vi "init.vi"(8 "error in (no error)":errorcluster, 11 "HP83712B_RF_Generator in":refnum<class "HP83712B_RF_Generator.lvclass">) -> (0 "error out":errorcluster, 3 "HP83712B_RF_Generator out":refnum<class "HP83712B_RF_Generator.lvclass">)   [LabVIEW 2013, in "HP83712B_RF_Generator.lvclass"]
uses:
  HP83712B_RF_Generator.lvclass
  HP83712B_RF_Generator.lvclass/HP83712B_RF_Generator.ctl
  Experiment/Globals.vi
  HP8662A_RF_Generator/HP8662A_RF_Generator.lvclass
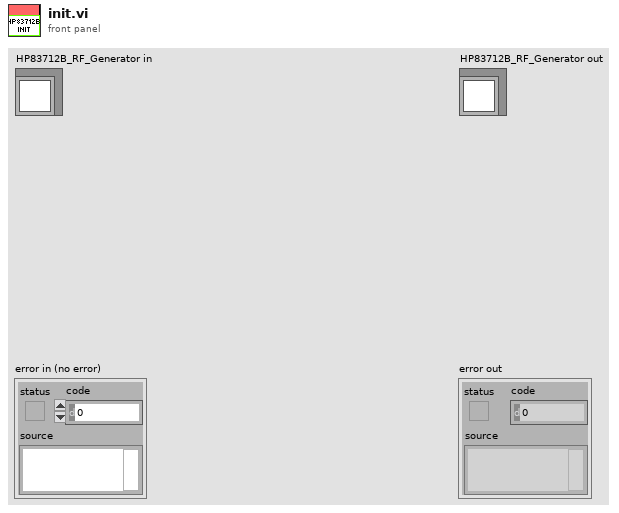
[diagram p1: front panel]
types:
  T1 = typedef "GPIB.lvclass/RF_Generator_settings_array.ctl" = T2[]
  T2 = typedef "GPIB.lvclass/RF_Generator_settings.ctl" = cluster{"Enable":bool, "Description":string, "GPIB channel #":u8, "Frequency (MHz)":dbl, "Power (dBm)":dbl}
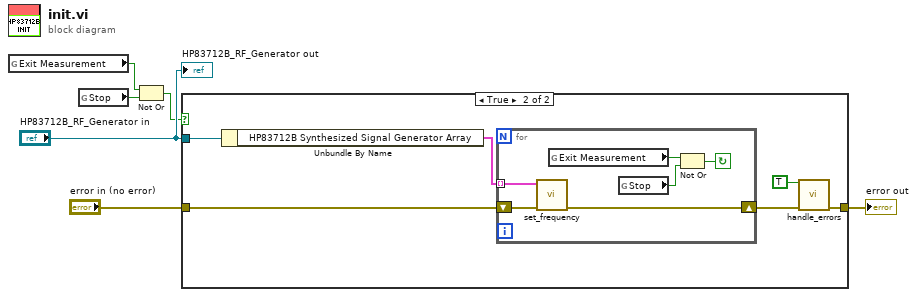
[diagram p0: block diagram]
diagram:
  n1 = global read "Globals.vi" "Exit Measurement"() -> (w3:bool)
  n2 = global read "Globals.vi" "Stop"() -> (w2:bool)
  n3 = Not Or(1:w2, 2:w3) -> (0:w1:bool)
  n4 = case shown="True" w1 {
    tunnel: "error in (no error)" -> [w7 w11]
    tunnel: [w7 w10] -> w5
    tunnel: "HP83712B_RF_Generator in" -> [_ w9]
    frame False {
    }
    frame True {
      n5 = Unbundle By Name(w9) -> ("HP83712B Synthesized Signal Generator Array"=w12:T1)
      n6 = for {
        tunnel: w12 -> [w19] mode=indexing
        shift-right: [w18] -> w13
        shift-left: w11 -> [w17]
        stop <- w14 continue-if-true
        n7 = call "set_frequency.vi"("error in"=w17, "RF Generator settings"=w19) -> ("error out"=w18:errorcluster)  [unwired: 9 in]
        n8 = global read "Globals.vi" "Exit Measurement"() -> (w16:bool)
        n9 = global read "Globals.vi" "Stop"() -> (w15:bool)
        n10 = Not Or(1:w15, 2:w16) -> (0:w14:bool)
      }
      n11 = call "handle_errors.vi"("Exit Operation"=TRUE, "error in (no error)"=w13) -> ("error out"=w10:errorcluster)  [unwired: 13 in]
    }
  }
  "error out" <- w5
  "HP83712B_RF_Generator out" <- "HP83712B_RF_Generator in"
